vi "Ev Apply.vi"(8 "error in (no error)":errorcluster, 11 "IDE simple in":refnum<class "Main Panel.lvclass">) -> (0 "error out":errorcluster, 3 "IDE simple out":refnum<class "Main Panel.lvclass">)   [LabVIEW 2018, in "Main Panel.lvlib" / "Main Panel.lvclass"]
uses:
  Main Panel.lvclass
  Main Panel.lvclass/Main Panel.ctl
  Frame Analizer/Data Parser.lvclass
  ScintillaNET/ScintillaNET.lvclass
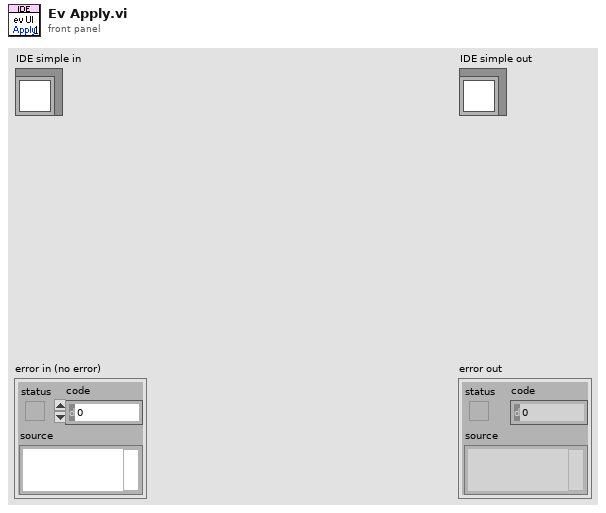
[diagram p1: front panel]
types:
  T1 = typedef "Data Parser.lvclass/frame data.ctl" = cluster{"Title":T2, "Basic Data":T3, "Sound":string, "<o> Data":T4, "<bp> Data":T5, "<c> Data":T6, "<w> Data":T7, "<i> Data Array":T8[], "<b> Data Array":T9[]}
  T2 = typedef "Data Parser.lvclass/frame title.ctl" = cluster{"Number":string, "Name":string}
  T3 = typedef "Data Parser.lvclass/frame basic data.ctl" = cluster{"Basic":cluster{"pic":string, "state":string, "wait":string, "next":string}, "Move":cluster{"dvx":string, "dvy":string, "dvz":string}, "Pic Center":cluster{"centerx":string, "centery":string}, "Skill":cluster{"hit_a":string, "hit_d":string, "hit_j":string, "hit_Fa":string, "hit_Ua":string, "hit_Da":string, "hit_Fj":string, "hit_Uj":string, "hit_Dj":string, "hit_ja":string}, "Mp":string}
  T4 = typedef "Data Parser.lvclass/frame o data.ctl" = cluster{"kind":string, "x":string, "y":string, "action":string, "dvx":string, "dvy":string, "dvz":string, "oid":string, "facing":string}
  T5 = typedef "Data Parser.lvclass/frame bp data.ctl" = cluster{"x":string, "y":string}
  T6 = typedef "Data Parser.lvclass/frame c data.ctl" = cluster{"kind":string, "x":string, "y":string, "injury":string, "cover":string, "vaction":string, "aaction":string, "taction":string, "hurtable":string, "decrease":string, "fronthurtact":string, "backhurtact":string, "dircontrol":string, "throwvx":string, "throwvy":string, "throwvz":string, "throwinjury":string}
  T7 = typedef "Data Parser.lvclass/frame w data.ctl" = cluster{"kind":string, "x":string, "y":string, "weaponact":string, "dvx":string, "dvy":string, "dvz":string, "attacking":string, "cover":string}
  T8 = typedef "Data Parser.lvclass/frame i data.ctl" = cluster{"kind":string, "x":string, "y":string, "w":string, "h":string, "dvx":string, "dvy":string, "dvz":string, "fall":string, "arest":string, "vrest":string, "bdefend":string, "injury":string, "zwidth":string, "effect":string, "catchingact":string, "caughtact":string}
  T9 = typedef "Data Parser.lvclass/frame b data.ctl" = cluster{"kind":string, "x":string, "y":string, "w":string, "h":string}
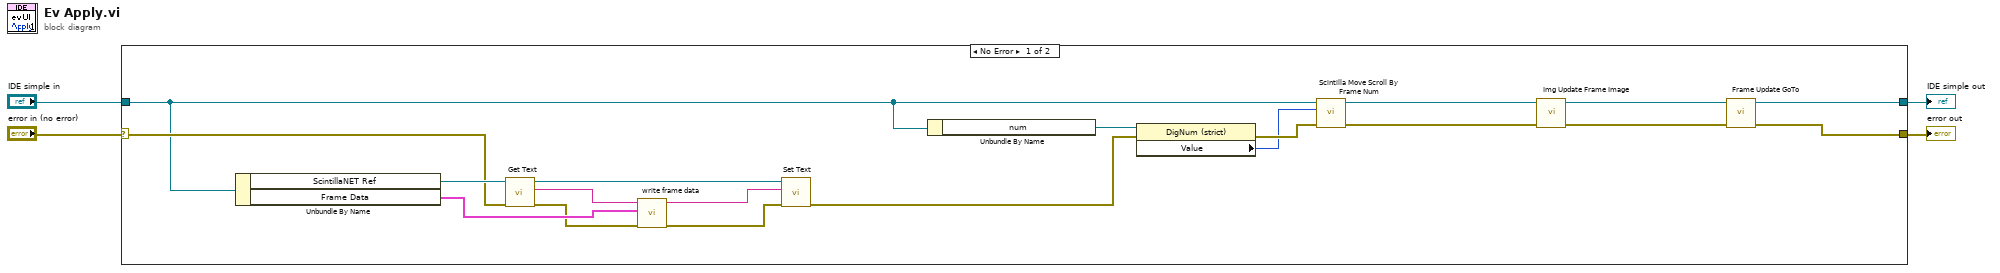
[diagram p0: block diagram]
diagram:
  n1 = case shown="No Error" "error in (no error)" {
    selector: "error in (no error)" -> [w16 w25]
    tunnel: [w9 w25] -> w3
    tunnel: [w10 w24] -> w1
    tunnel: "IDE simple in" -> [w14 w24]
    frame No Error {
      n2 = Unbundle By Name(w14) -> ("ScintillaNET Ref"=w22:refnum<class "ScintillaNET.lvclass">, "Frame Data"=w23:T1)
      n3 = call "Get Text.vi"("error in (no error)"=w16, "ScintillaNET in"=w22) -> ("error out"=w20:errorcluster, "Text"=w21:string, "ScintillaNET out"=w18:refnum<class "ScintillaNET.lvclass">)  [unwired: 7 in]
      n4 = call "write frame data.vi"("error in"=w20, "frame data"=w23, "file string in"=w21) -> ("error out"=w19:errorcluster, "file string out"=w17:string)  [unwired: 7 in]
      n5 = call "Set Text.vi"("error in (no error)"=w19, "Text"=w17, "ScintillaNET in"=w18) -> ("error out"=w13:errorcluster)  [unwired: 7 in, 1 out]
      n6 = Unbundle By Name(w14) -> ("num"=w15:refnum<vi>)
      n7 = property class="DigNum (strict)"(reference=w15, error in=w13) -> (error out=w12:errorcluster, "Value"=w11:u32)  [unwired: 1 out]
      n8 = call "Scintilla Move Scroll By Frame Num.vi"("error in (no error)"=w12, "Frame Number"=w11, "IDE simple in"=w14) -> ("error out"=w7:errorcluster, "IDE simple out"=w8:refnum<class "Main Panel.lvclass">)  [unwired: 7 in]
      n9 = call "Img Update Frame Image.vi"("error in (no error)"=w7, "LF2R IDE in"=w8) -> ("error out"=w5:errorcluster, "LF2R IDE out"=w6:refnum<class "Main Panel.lvclass">)  [unwired: 8 in]
      n10 = call "Frame Update GoTo.vi"("error in (no error)"=w5, "LF2R IDE in"=w6) -> ("error out"=w9:errorcluster, "LF2R IDE out"=w10:refnum<class "Main Panel.lvclass">)  [unwired: 8 in]
    }
    frame Error {
    }
  }
  "error out" <- w3
  "IDE simple out" <- w1
